vi "CSTK_MCListbox_Designer_ModiifyColHdrsAttrBatches.vi"(8 "错误输入（无错误）":errorcluster, 9 "Attr":T1[](array[typedef]), 10 "MulticolumnListbox输入":refnum<vi>, 11 "VI输入":refnum<vi>) -> (0 "错误输出":errorcluster, 3 "VI输出":refnum<vi>)   [LabVIEW 2015, in "CSTK_MCListbox Designer.lvlib"]
uses:
  CSTK_MCListbox Designer.lvlib
  _CSTK_MCListbox_Designer_ColHdr_Selected.ctl
  _CSTK_MCListbox_Designer_ColHdr.ctl
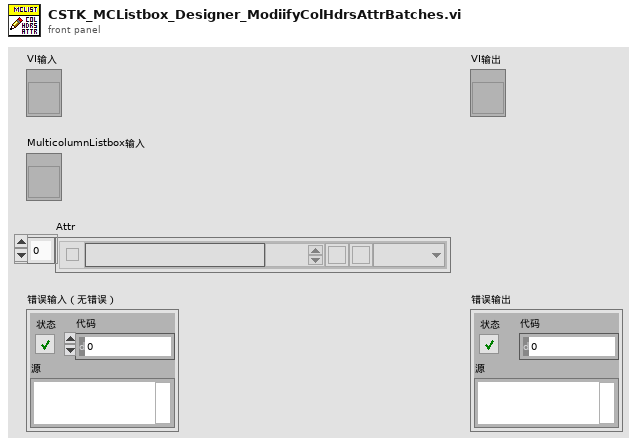
[diagram p1: front panel]
types:
  T1 = typedef "CSTK_MCListbox Designer.lvlib/_CSTK_MCListbox_Designer_ColHdr_Selected.ctl" = cluster{"选择":bool, "表头属性":T2}
  T2 = typedef "CSTK_MCListbox Designer.lvlib/_CSTK_MCListbox_Designer_ColHdr.ctl" = cluster{"列名称":string, "单元格宽度":u32, "粗体":bool, "斜体":bool, "对齐":enum16{"Left", "Center", "Right"}}
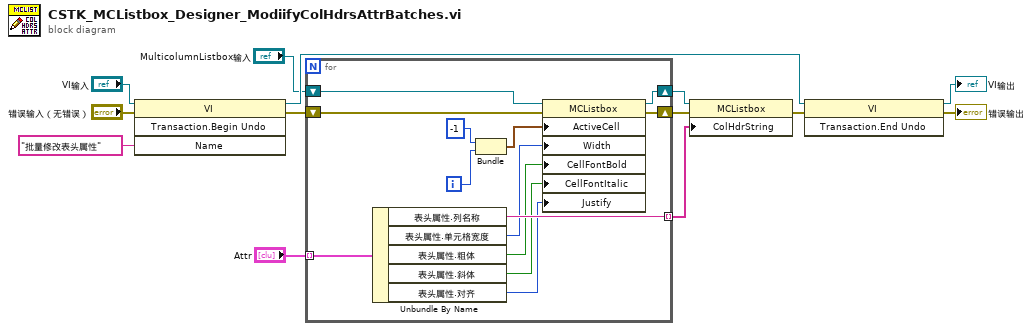
[diagram p0: block diagram]
diagram:
  n1 = invoke class="VI" method="Transaction.Begin Undo"(reference="VI输入", error in="错误输入（无错误）", "Name"="批量修改表头属性" ("名称")) -> (reference out=w11:refnum<vi>, error out=w9:errorcluster)  [unwired: 1 in, 2 out]
  n2 = for {
    tunnel: "Attr" -> [w24] mode=indexing
    tunnel: [w23] -> w2 mode=indexing
    shift-right: [w20] -> w1
    shift-left: "MulticolumnListbox输入" -> [w21]
    shift-right: [w15] -> w4
    shift-left: w9 -> [w16]
    i -> [w25]
    n3 = Unbundle By Name(w24) -> ("表头属性.列名称"=w23:string, "表头属性.单元格宽度"=w19:u32, "表头属性.粗体"=w18:bool, "表头属性.斜体"=w14:bool, "表头属性.对齐"=w17:enum16{"Left", "Center", "Right"})
    n4 = Bundle(-1, w25) -> (w22:cluster{i32, i32})  [unwired: 1 in]
    n5 = property class="MCListbox"(reference=w21, error in=w16, "ActiveCell"=w22, "Width"=w19, "CellFontBold"=w18, "CellFontItalic"=w14, "Justify"=w17) -> (reference out=w20:refnum<vi>, error out=w15:errorcluster)
  }
  n6 = property class="MCListbox"(reference=w1, error in=w4, "ColHdrString"=w2) -> (error out=w10:errorcluster)  [unwired: 1 out]
  n7 = invoke class="VI" method="Transaction.End Undo"(reference=w11, error in=w10) -> (reference out=→"VI输出":refnum<vi>, error out=→"错误输出":errorcluster)  [unwired: 1 in, 1 out]
